vi "TriggerRotationInitAcquire.vi"(0 "Microscope in":refnum<class "Microscope.lvclass">, 5 "TabName":string="TabControl", 7 "Page":i32=1, 9 "Control Name":string="Initialize AngleScan", 11 "error in (no error)":errorcluster, 12 "relative vi path":string="RotationProgram\\RotationApplication.vi") -> (4 "Microscope out":refnum<class "Microscope.lvclass">, 15 "error out":errorcluster)   [LabVIEW 2012, in "Microscope.lvclass"]
uses:
  classes/Microscope.lvclass
  classes/Microscope.lvclass/Microscope.ctl
  RotationProgram/Event/MainEvents.ctl
  RotationProgram/Global/RotationGlobal.vi
panel:
  out "VI out":refnum<vi>
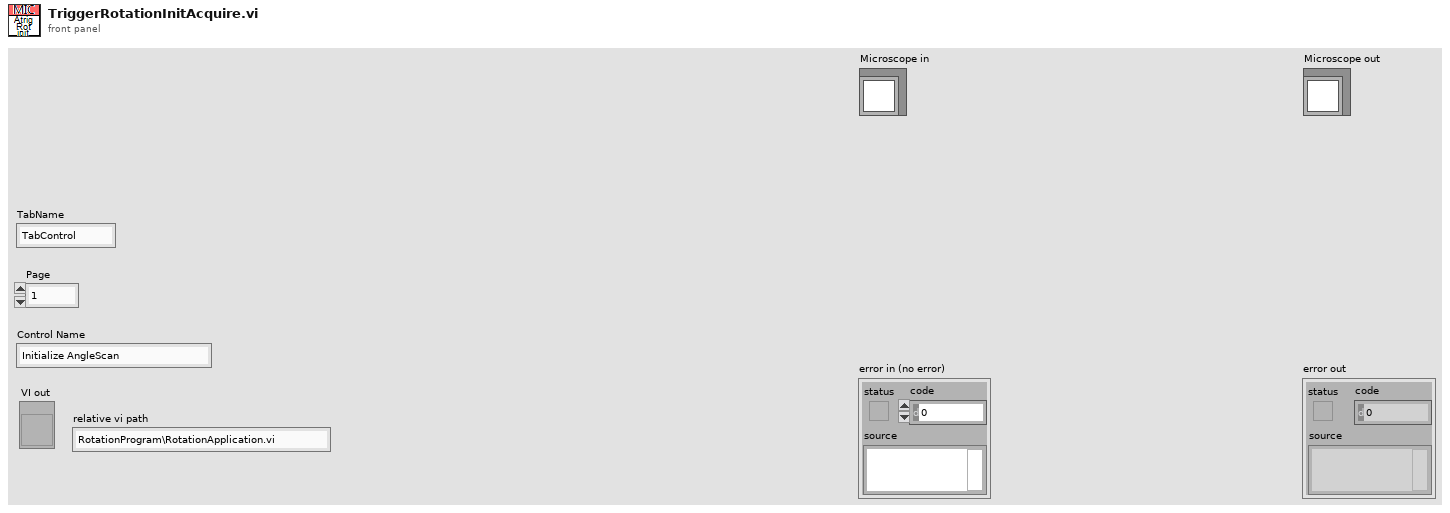
[diagram p1: front panel]
types:
  T1 = typedef "MainEvents.ctl" = enum16{"Initialize", "Initialize Angle Scan", "Acquire Angle Scan", "Move to Zero", "Home", "Send Request", "Move Relative Negative", "Move Relative", "Optimize", "Move Absolute", "Calibrate Angle-Stage", "Restore Sync Parameters", "Sync Formula", "Sync Data", "Sync Data Shotgun", "Restore Booleans", "Disable Buttons", "Enable Buttons"}
  T2 = typedef "ScanMode.ctl" = enum16{"None", "Continuous", "Point Scan (CH3 cursor)", "Point Scan Move (CH3 cursor)", "Grab", "Grab Move Stage", "Grab Move Z-stage", "Cont. Move Z-stage", "Spec Move Stage", "Spec Move Cont", "Surf Calib"}
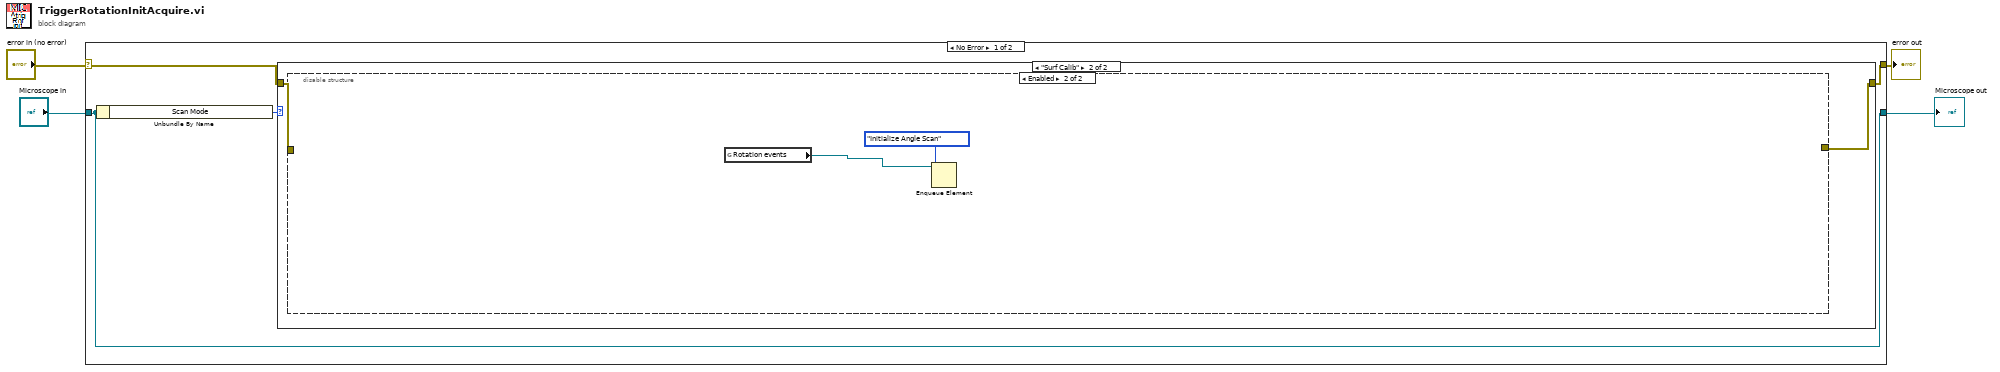
[diagram p0: block diagram]
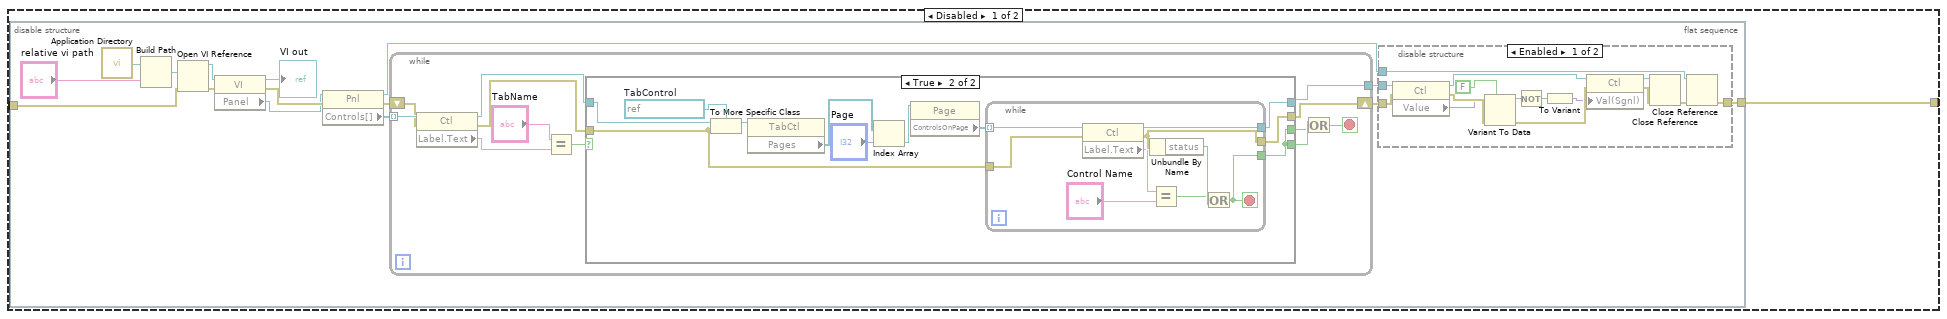
[diagram p3: hidden frame]
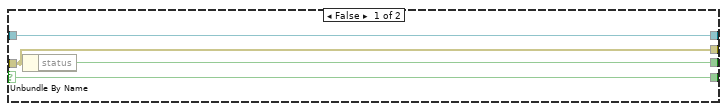
[diagram p5: hidden frame]
diagram:
  n1 = case shown="No Error" "error in (no error)" {
    selector: "error in (no error)" -> [w6 w83]
    tunnel: [w7 w83] -> w3
    tunnel: [w8 w82] -> w1
    tunnel: "Microscope in" -> [w8 w82]
    frame No Error {
      n2 = Unbundle By Name(w8) -> ("Scan Mode"=w5:T2)
      n3 = case shown="\"Surf Calib\"" w5 {
        tunnel: [w9 w11] -> w7
        tunnel: w6 -> [w9 w10]
        frame "None", Default {
        }
        frame "Surf Calib" {
          n4 = disable-structure shown="Enabled" {
            disable-tunnel: [w13 _] -> w11
            disable-tunnel: w10 -> [w12 _]
            frame Disabled {
              n5 = flat-sequence {
                tunnel: [w15] -> w13
                tunnel: w12 -> [w14]
                frame #0 {
                  n6 = call <vilib>:"Application Directory.vi"() -> ("Application Directory"=w20:path)
                  n7 = Build Path(base path=w20, name or relative path="relative vi path") -> (appended path=w19:path)
                  n8 = Open VI Reference(vi path=w19, error in (no error)=w14) -> (vi reference=w18:refnum<vi>, error out=w17:errorcluster)  [unwired: 4 in]
                  n9 = property class="VI"(reference=w18, error in=w17) -> (reference out=→"VI out":refnum<vi>, error out=w25:errorcluster, "Panel"=w21:refnum<vi>)
                  n10 = property class="Pnl"(reference=w21, error in=w25) -> (reference out=w28:refnum<vi>, error out=w26:errorcluster, "Controls[]"=w22:refnum<vi>[])
                  n11 = while {
                    tunnel: w22 -> [w55] mode=indexing
                    tunnel: [w52] -> w23
                    shift-right: [w47] -> w27
                    shift-left: w26 -> [w53]
                    stop <- w49 stop-if-true
                    n12 = property class="Ctl"(reference=w55, error in=w53) -> (reference out=w45:refnum<vi>, error out=w48:errorcluster, "Label.Text"=w54:string)
                    n13 = Equal?(x="TabName", y=w54) -> (x = y?=w51:bool)
                    n14 = case shown="True" w51 {
                      selector: w51 -> [w59 _]
                      tunnel: [w56 w70] -> w52
                      tunnel: [w59 w60] -> w50
                      tunnel: w48 -> [w57 w65]
                      tunnel: [w57 w69] -> w47
                      tunnel: w45 -> [w56 w66]
                      tunnel: [w58 w60] -> w44
                      frame False {
                        n15 = Unbundle By Name(w57) -> ("status"=w58:bool)
                      }
                      frame True {
                        w67 = refnum<vi> refnum  # TabControl
                        n16 = To More Specific Class(target class=w67, reference=w66, error in=w65) -> (specific class reference=w64:refnum<vi>)  [unwired: 1 out]
                        n17 = property class="TabCtl"(reference=w64) -> ("Pages"=w63:refnum<vi>[])  [unwired: 1 in, 2 out]
                        n18 = Index Array(array=w63, index="Page") -> (element=w62:refnum<vi>)
                        n19 = property class="Page"(reference=w62) -> ("ControlsOnPage"=w61:refnum<vi>[])  [unwired: 1 in, 2 out]
                        n20 = while {
                          tunnel: [w79] -> w70
                          tunnel: [w76] -> w60
                          tunnel: w65 -> [w75]
                          tunnel: [w74] -> w69
                          tunnel: w61 -> [w71] mode=indexing
                          stop <- w76 stop-if-true
                          n21 = property class="Ctl"(reference=w71, error in=w75) -> (reference out=w79:refnum<vi>, error out=w74:errorcluster, "Label.Text"=w73:string)
                          n22 = Unbundle By Name(w74) -> ("status"=w78:bool)
                          n23 = Equal?(x=w73, y="Control Name") -> (x = y?=w77:bool)
                          n24 = Or(x=w77, y=w78) -> (x .or. y?=w76:bool)
                        }
                      }
                    }
                    n25 = Or(x=w50, y=w44) -> (x .or. y?=w49:bool)
                  }
                  n26 = disable-structure shown="Enabled" {
                    disable-tunnel: w28 -> [w43 _]
                    disable-tunnel: w27 -> [w39 _]
                    disable-tunnel: w23 -> [w30 _]
                    disable-tunnel: [w29 _] -> w15
                    frame Enabled {
                      n27 = property class="Ctl"(reference=w30, error in=w39) -> (reference out=w31:refnum<vi>, error out=w37:errorcluster, "Value"=w33:variant)
                      n28 = Variant To Data(error in=w37, type=FALSE ("Push Other VI's Button 2"), Variant=w33) -> (data=w36:bool, error out=w38:errorcluster)
                      n29 = Not(x=w36) -> (.not. x?=w35:bool)
                      n30 = To Variant(anything=w35) -> (Variant=w32:variant)
                      n31 = property class="Ctl"(reference=w31, error in=w38, "Val(Sgnl)"=w32) -> (reference out=w42:refnum<vi>, error out=w41:errorcluster)
                      n32 = Close Reference(reference=w42, error in (no error)=w41) -> (error out=w40:errorcluster)
                      n33 = Close Reference(reference=w43, error in (no error)=w40) -> (error out=w29:errorcluster)
                    }
                    frame Disabled {
                    }
                  }
                }
              }
            }
            frame Enabled {
              n34 = global read "RotationGlobal.vi" "Rotation events"() -> (w80:refnum<queue>)
              n35 = Enqueue Element(queue=w80, element=MainEvents."Initialize Angle Scan") -> ()  [unwired: 2 in, 3 out]
            }
          }
        }
      }
    }
    frame Error {
    }
  }
  "error out" <- w3
  "Microscope out" <- w1
